vi "Vision-Target.vi"(8 "error in (no error)":errorcluster, 11 "Image Size":T5=enum."320x240") -> ()   [LabVIEW 2019]
uses:
  <vilib>/Rock Robotics/WPI/Camera/WPI_CameraImageSize.ctl
  vision/Camera Types.ctl
  <vilib>/Rock Robotics/WPI/Camera/WPI_CameraWhite Balance Values.ctl
  <vilib>/Rock Robotics/WPI/Camera/WPI_CameraExposure Values.ctl
  <vilib>/Rock Robotics/WPI/Camera/WPI_CameraFrameRate.ctl
  Robot Global Data.vi
  <vilib>/vision/NI_Vision_Development_Module.lvlib
panel:
  out "Angle":dbl
  out "Speed":dbl
  out "Possible":bool
  out "Disqualified":i32
  out "Results":T1(array[cluster]) {"Normalized Center"."x" format="%#_2g"; "Normalized Center"."y" format="%#_2g"; "Overall Score" format="%#_2g"; "Distance (ft)" format="%#_3g"; "Area Score" format="%#_2g"; "Moment Score" format="%#_2g"; "Aspect Score" format="%#_2g"}
  in  "Size Limit %":dbl=0.04 min=0.0 max=100.0 step=0.01 format="%#_13g"
  in  "Color Mode":u16(ring)=2 items=["RGB", "HSL", "HSV", "HSI"]
  in  "Particle Count":i32=5
  in  "Score Threshold %":dbl=75.0
  in  "Std Devs for Calibration":cluster{"H":dbl, "S":dbl, "V":dbl}={"H"=4.0, "S"=8.0, "V"=8.0}
  in  "Camera Type (for distance)":T2=enum."MS HD3000 square"
  in  "Annotate":bool=TRUE
  out "Qualified":i32
  in  "LED Color Range":T3={"Hue"={92.46666717529297, 124.46666717529297}, "Sat"={154.82142857142856, 255.0}, "Val"={100.17857142857144, 251.32874298095703}} {"Hue" scale=0.0..255.0 scale format="%#_3g"}
  out "Mask":T4(plugin-control)
  out "Original Image":T4(plugin-control)
  out "loop ms":u32
  out "Instructions:":string="Connect a USB or IP camera to your roboRIO. If using a ring light and retroreflective tape, use Camera Settings outside the loop create a dark image with bright and colorful stripes. If used wihtout a ring light, brighten the images so that stripes are visible.\n\nLED Color can encoded as HSL or related color modes. Calibrate to the same color as the strips being reflected to the camera. Unlike the desktop example, this LED color must be set by hand. You can also put the calibration on the dashboard and send the LED Color to the RT code using Network Tables.\n\nThe Display buttons affects whether images are displayed on the panel. It takes quite a bit of CPU  to compress and transmit the images for display.\n\nAdjust Score Cutoff to make the code more or less picky. If the color is not very unique, you may need to increase the number of particles considered. The diagram uses a Size Limit to ignore colored things that are too small. You may need to adjust it if you are targetting from far away.\n\nResults give you the distance to the target, the center and box in a normalized (-1 to 1) and pixel coordinates.\n\nBe sure to read about setting camera exposure and brightness to help simplify your image and acquire color saturated images.\n\nThere are lots of comments on the diagram to explain the code."
  # "Scores"
  # "Good target, distance ft"
  # "Bad target"
  # "Score in %"
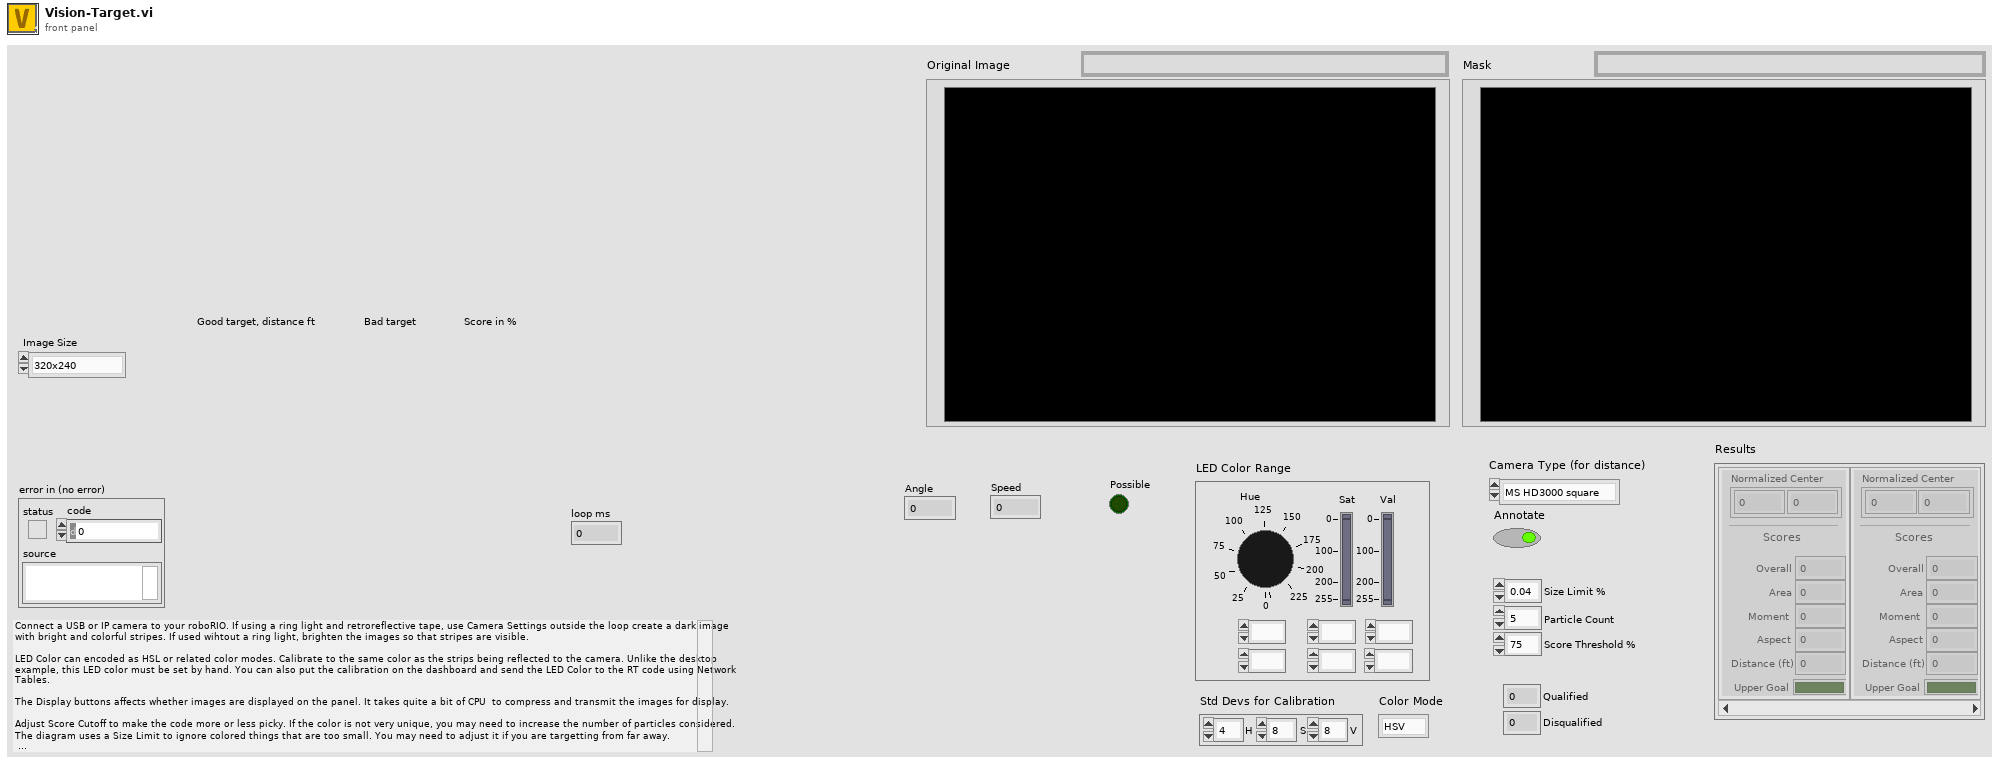
[diagram p1: front panel]
types:
  T1 = cluster{"diameter points":cluster{"first point":cluster{"x":dbl, "y":dbl}, "projected point":cluster{"x":dbl, "y":dbl}}, "Normalized Center":cluster{"x":dbl, "y":dbl}, "Overall Score":dbl, "Area Score":dbl, "Moment Score":dbl, "Aspect Score":dbl, "Distance (ft)":dbl, "Upper Goal":bool}[]
  T2 = typedef "Camera Types.ctl" = enum16{"206", "1011", "1013", "MS HD3000 square", "MS HD3000 640x480"}
  T3 = cluster{"Hue":cluster{dbl, dbl}, "Sat":cluster{dbl, dbl}, "Val":cluster{dbl, dbl}}
  T4 = typedef "IMAQ Image.ctl" = refnum<image>
  T5 = typedef "WPI_CameraImageSize.ctl" = enum16{"640x480", "320x240", "160x120", "Custom"}
  T6 = typedef "Particle Parameters" = i32
  T7 = typedef "WPI_CameraFrameRate.ctl" = u32
  T8 = typedef "WPI_CameraExposure Values.ctl" = enum16{"Auto", "Flicker-free 50 Hz", "Flicker-free 60 Hz", "Hold current", "Custom"}
  T9 = typedef "WPI_CameraWhite Balance Values.ctl" = enum16{"Auto", "Fixed indoor", "Fixed outdoor 1", "Fixed outdoor 2", "Fixed fluorescent 1", "Fixed fluorescent 2", "Hold current", "Custom"}
  T10 = typedef "Image Type" = u32
  T11 = typedef "WPI_CameraDevRef.ctl" = cluster{"Camera Address":string, "CameraStatus":errorcluster}
  T12 = enum32{"AutoM", "Close", "Dilate", "Erode", "Gradient", "Gradient out", "Gradient in", "Hit miss", "Open", "PClose", "POpen", "Thick", "Thin"}
  T13 = cluster{cluster{dbl, dbl}, cluster{dbl, dbl}, cluster{dbl, dbl}}
  T14 = cluster{"remainder":i32, "size":bool, "count":bool}
  T15 = typedef "Target Fields.ctl" = cluster{"diameter points":cluster{"first point":cluster{"x":dbl, "y":dbl}, "projected point":cluster{"x":dbl, "y":dbl}}, "normalized center":cluster{"x":dbl, "y":dbl}, "Overall Score":dbl, "Area Score":dbl, "Moment Score":dbl, "Aspect Score":dbl, "Distance (ft)":dbl, "Upper Goal":bool}
  T16 = cluster{"[0]":T15, "[1]":T15, "[2]":T15, "[3]":T15, "[4]":T15, "[5]":T15, "[6]":T15, "[7]":T15, "[8]":T15}
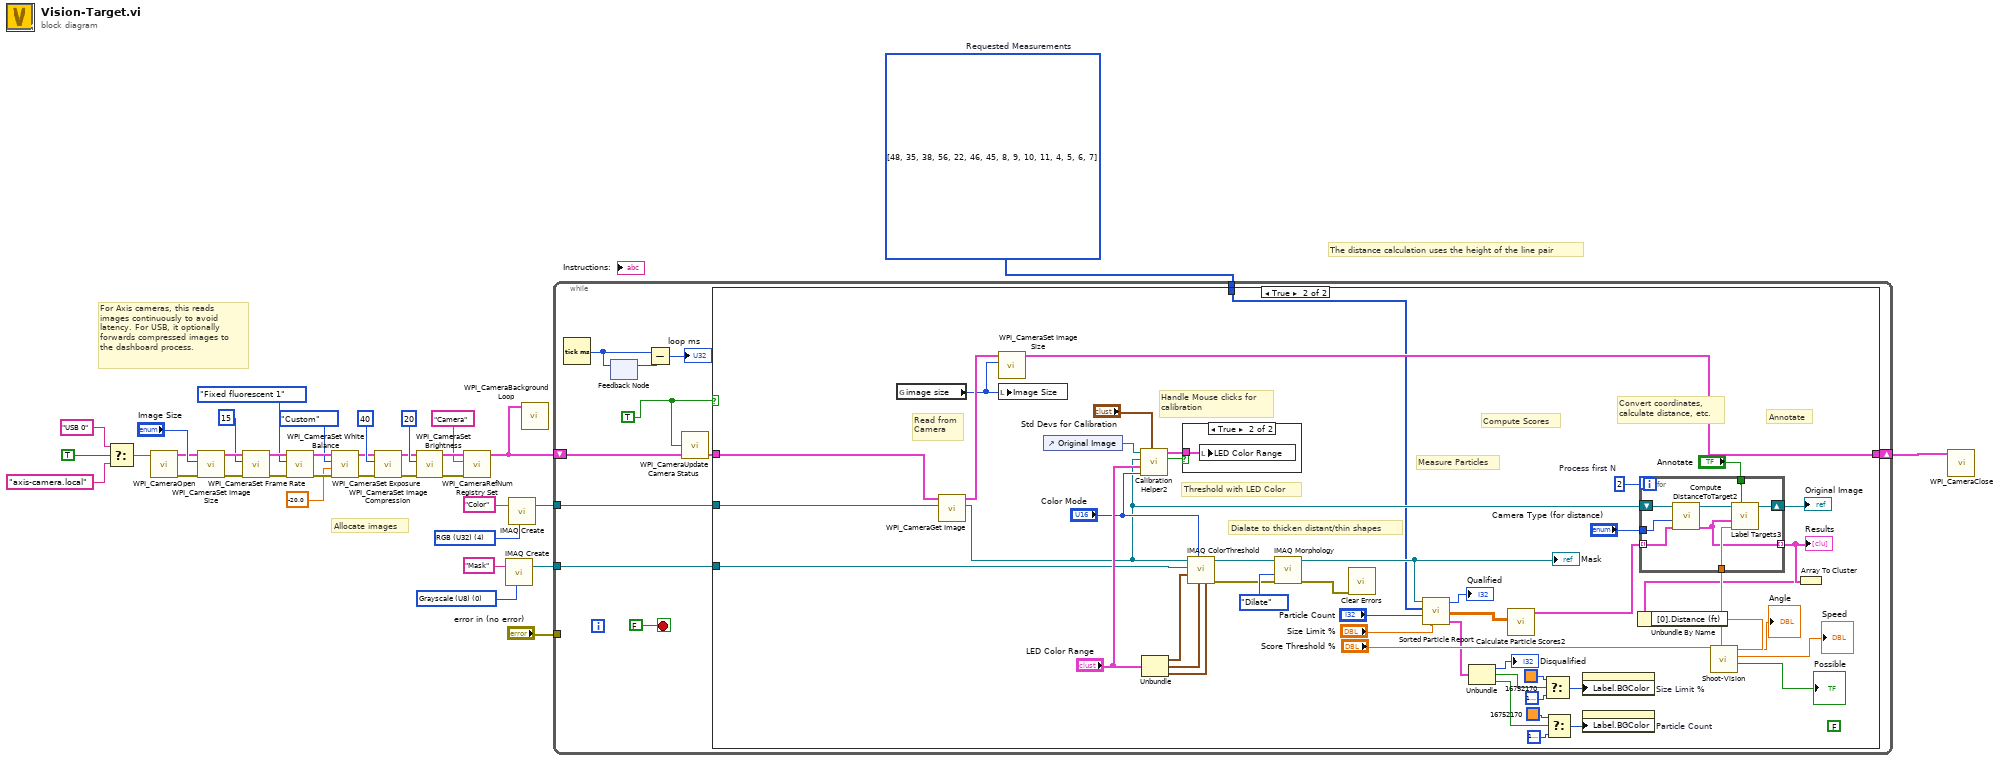
[diagram p0: block diagram]
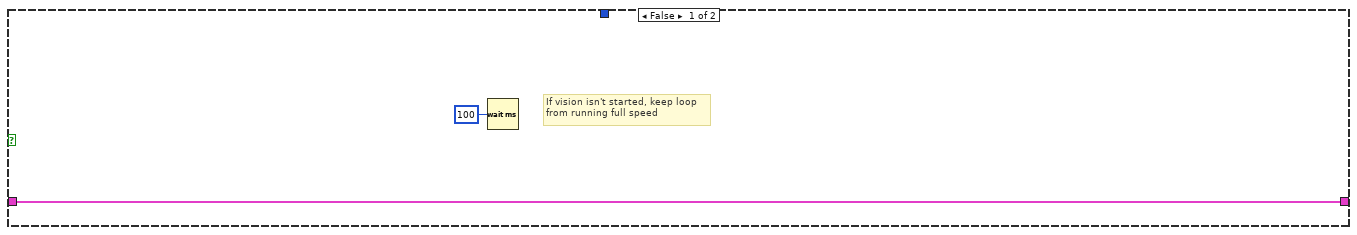
[diagram p2: hidden frame]
diagram:
  w1 = T6[] [48, 35, 38, 56, 22, 46, 45, 8, 9, 10, 11, 4, 5, 6, 7] items=["Center of Mass X", "Center of Mass Y", "First Pixel X", "First Pixel Y", "Bounding Rect Left", "Bounding Rect Top", "Bounding Rect Right", "Bounding Rect Bottom", "Max Feret Diameter Start X", "Max Feret Diameter Start Y", "Max Feret Diameter End X", "Max Feret Diameter End Y", "Max Horiz. Segment Length Left", "Max Horiz. Segment Length Right", "Max Horiz. Segment Length Row", "-", "Bounding Rect Width", "Bounding Rect Height", "Bounding Rect Diagonal", "Perimeter", "Convex Hull Perimeter", "Holes' Perimeter", "Max Feret Diameter", "Equivalent Ellipse Major Axis", "Equivalent Ellipse Minor Axis", "Equivalent Ellipse Minor Axis (Feret)", "Equivalent Rect Long Side", "Equivalent Rect Short Side", "Equivalent Rect Diagonal", "Equivalent Rect Short Side (Feret)", "Average Horiz. Segment Length", "Average Vert. Segment Length", "Hydraulic Radius", "Waddel Disk Diameter", "-", "Area", "Holes' Area", "Particle & Holes' Area", "Convex Hull Area", "Image Area", "-", "Number of Holes", "Number of Horiz. Segments", "Number of Vert. Segments", "-", "Orientation", "Max Feret Diameter Orientation", "-", "% Area/Image Area", "% Area/(Particle & Holes' Area)", "Ratio of Equivalent Ellipse Axes", "Ratio of Equivalent Rect Sides", "-", "Elongation Factor", "Compactness Factor", "Heywood Circularity Factor", "Type Factor", "-", "Sum X", "Sum Y", "Sum XX", "Sum XY", "Sum YY", "Sum XXX", "Sum XXY", "Sum XYY", "Sum YYY", "-", "Moment of Inertia XX", "Moment of Inertia XY", "Moment of Inertia YY", "Moment of Inertia XXX", "Moment of Inertia XXY", "Moment of Inertia XYY", "Moment of Inertia YYY", "Norm. Moment of Inertia XX", "Norm. Moment of Inertia XY", "Norm. Moment of Inertia YY", "Norm. Moment of Inertia XXX", "Norm. Moment of Inertia XXY", "Norm. Moment of Inertia XYY", "Norm. Moment of Inertia YYY", "Hu Moment 1", "Hu Moment 2", "Hu Moment 3", "Hu Moment 4", "Hu Moment 5", "Hu Moment 6", "Hu Moment 7"]  # Requested Measurements
  w34 = T10 0 items=["Grayscale (U8)", "Grayscale (I16)", "Grayscale (SGL)", "Complex (CSG)", "RGB (U32)", "HSL (U32)", "RGB (U64)", "Grayscale (U16)"] ("Image Type")
  w35 = T10 4 items=["Grayscale (U8)", "Grayscale (I16)", "Grayscale (SGL)", "Complex (CSG)", "RGB (U32)", "HSL (U32)", "RGB (U64)", "Grayscale (U16)"] ("Image Type")
  # "For Axis cameras, this reads\nimages continuously to avoid\nlatency. For USB, it optionally\nforwards compressed images to\nthe dashboard process."
  # "The distance calculation uses the height of the line pair"
  # "Allocate images"
  n1 = Select(t="USB 0" ("format string"), s=TRUE ("dot notation? (F)"), f="axis-camera.local" ("format string")) -> (s? t:f=w6:string)
  n2 = call <vilib>:"WPI_CameraOpen.vi"("Camera Address"=w6) -> ("error out"=w18:errorcluster, "CameraDevRef"=w19:T11)  [unwired: 1 in, 8 out]
  n3 = call <vilib>:"WPI_CameraSet Image Size.vi"("error in (no error)"=w18, "Image Size"="Image Size", "CameraDevRef"=w19) -> ("error out"=w17:errorcluster, "CameraDevRef Out"=w20:T11)  [unwired: 1 in, 6 out]
  n4 = call <vilib>:"WPI_CameraSet Frame Rate.vi"("error in (no error)"=w17, "Frame Rate (fps)"=T7 15, "CameraDevRef"=w20) -> ("error out"=w16:errorcluster, "CameraDevRef Out"=w22:T11)  [unwired: 7 out]
  n5 = call <vilib>:"WPI_CameraSet White Balance.vi"("error in (no error)"=w16, "White Balance"=WPI_CameraWhite_Balance_Values."Fixed fluorescent 1", "CameraDevRef"=w22) -> ("error out"=w15:errorcluster, "CameraDevRef Out"=w21:T11)  [unwired: 1 in, 6 out]
  n6 = call <vilib>:"WPI_CameraSet Exposure.vi"("error in (no error)"=w15, "Exposure (%)"=-20.0, "Exposure"=WPI_CameraExposure_Values."Custom", "CameraDevRef"=w21) -> ("error out"=w14:errorcluster, "CameraDevRef Out"=w24:T11)  [unwired: 6 out]
  n7 = call <vilib>:"WPI_CameraSet Image Compression.vi"("error in (no error)"=w14, "Compression"=40, "CameraDevRef"=w24) -> ("error out"=w13:errorcluster, "CameraDevRef Out"=w23:T11)  [unwired: 7 out]
  n8 = call <vilib>:"WPI_CameraSet Brightness.vi"("error in (no error)"=w13, "Brightness"=20, "CameraDevRef"=w23) -> ("error out"=w12:errorcluster, "CameraDevRef Out"=w30:T11)  [unwired: 1 in, 6 out]
  n9 = call <vilib>:"WPI_CameraRefNum Registry Set.vi"("error in (no error)"=w12, "refnum name"="Camera", "CameraDevRef"=w30) -> ("CameraDevRef"=w5:T11)  [unwired: 1 in, 7 out]
  n10 = call "IMAQ Create"("Image Name"="Mask", "Image Type"=w34) -> ("New Image"=w32:T4)  [unwired: 2 in, 2 out]
  n11 = call "IMAQ Create"("Image Name"="Color", "Image Type"=w35) -> ("New Image"=w31:T4)  [unwired: 2 in, 2 out]
  n12 = call <vilib>:"WPI_CameraBackground Loop.vi"("CameraDevRef"=w5) -> ()  [unwired: 11 in]
  n13 = while {
    tunnel: w31 -> [w44]
    tunnel: w32 -> [w46]
    tunnel: w1 -> [w45]
    shift-right: [w43] -> w4
    shift-left: w5 -> [w42]
    tunnel: "error in (no error)" -> [_]
    stop <- FALSE stop-if-true
    w37 = TRUE
    n14 = Tick Count (ms)() -> (millisecond timer value=w39:u32)
    n15 = feedback #1() -> (w40:u32)  [unwired: 1 in]
    n16 = feedback-in #1(w39) -> ()
    n17 = Subtract(x=w39, y=w40) -> (x-y=→"loop ms":u32)
    n18 = call <vilib>:"WPI_CameraUpdate Camera Status.vi"("CameraDevRef In"=w42, "Enable Vision"=w37) -> ("CameraDevRef Out"=w41:T11)  [unwired: 3 in]
    n19 = case shown="True" w37 {
      tunnel: w46 -> [_ w56]
      tunnel: w45 -> [_ w57]
      tunnel: w41 -> [w49 w97]
      tunnel: w44 -> [_ w96]
      tunnel: [w49 w93] -> w43
      frame False {
        # "If vision isn't started, keep loop\nfrom running full speed"
        n20 = Wait (ms)(milliseconds to wait=u32 100) -> ()  [unwired: 1 out]
      }
      frame True {
        w77 = 2  # Process first N
        (unwired) FALSE
        # "Dialate to thicken distant/thin shapes"
        # "Handle Mouse clicks for\ncalibration"
        # "Measure Particles"
        # "Convert coordinates,\ncalculate distance, etc."
        # "Annotate"
        # "Compute Scores"
        # "Threshold with LED Color"
        # "Read from\nCamera"
        n21 = global read "Robot Global Data.vi" "image size"() -> (w94:T5)
        n22 = call <vilib>:"WPI_CameraGet Image.vi"("Image"=w96, "CameraDevRef"=w97) -> ("Image Out"=w58:T4, "CameraDevRef Out"=w95:T11)  [unwired: 7 in, 1 out]
        n23 = call <vilib>:"WPI_CameraSet Image Size.vi"("Image Size"=w94, "CameraDevRef"=w95) -> ("CameraDevRef Out"=w93:T11)  [unwired: 2 in, 7 out]
        n24 = local write "Image Size"(w94) -> ()
        n25 = control-ref of="Original Image"() -> (w87:refnum<vi>)
        n26 = call "Calibration Helper2.vi"("Std Devs"="Std Devs for Calibration", "Color Mode"="Color Mode", "Color Components"="LED Color Range", "Image"=w58, "Image Ctl Refnum"=w87) -> ("Changed"=w86:bool, "output color"=w85:T13)  [unwired: 5 in]
        n27 = Unbundle("LED Color Range") -> ("Hue"=w92:cluster{dbl, dbl}, "Sat"=w91:cluster{dbl, dbl}, "Val"=w90:cluster{dbl, dbl})
        n28 = case shown="True" w86 {
          tunnel: w85 -> [_ w106]
          frame False {
          }
          frame True {
            n29 = local write "LED Color Range"(w106) -> ()
          }
        }
        n30 = call "IMAQ ColorThreshold"("Blue or Luma or Val or Inten Range"=w90, "Green or Sat Range"=w91, "Color Mode"="Color Mode", "Red or Hue Range"=w92, "Image Dst"=w56, "Image Src"=w58) -> ("error out"=w74:errorcluster, "Image Dst Out"=w76:T4)  [unwired: 4 in]
        n31 = call "IMAQ Morphology"("error in (no error)"=w74, "Operation"=T12."Dilate", "Image Src"=w76) -> ("error out"=w73:errorcluster, "Image Dst Out"=w70:T4)  [unwired: 7 in]
        "Mask" <- w70
        n32 = call <vilib>:"Clear Errors.vi"("error in (no error)"=w73) -> ()  [unwired: 5 in, 2 out]
        n33 = call "Sorted Particle Report.vi"("Min Area Size %"="Size Limit %", "Particle Count Limit"="Particle Count", "Pixel Measurements"=w57, "Image in"=w70) -> ("limits"=w68:T14, "Sorted Data"=w72:dbl[][], "Particles"=→"Qualified":i32)
        n34 = Unbundle(w68) -> ("remainder"=→"Disqualified":i32, "size"=w62:bool, "count"=w61:bool)
        n35 = call "Calculate Particle Scores2.vi"("Sorted Data"=w72) -> ("Scores"=w71:T15[])  [unwired: 10 in]
        n36 = Select(t=u32 16752170 ("Color"), s=w62, f=u32 16777216 ("Color")) -> (s? t:f=w60:u32)
        n37 = Select(t=u32 16752170 ("Color"), s=w61, f=u32 16777216 ("Color")) -> (s? t:f=w59:u32)
        n38 = property on="Size Limit %" class="DigNum (strict)"("Label.BGColor"=w60) -> ()  [unwired: 2 in, 2 out]
        n39 = property on="Particle Count" class="DigNum (strict)"("Label.BGColor"=w59) -> ()  [unwired: 2 in, 2 out]
        n40 = for {
          N: w77 -> [_]
          tunnel: w71 -> [w103] mode=indexing
          tunnel: "Camera Type (for distance)" -> [w105]
          tunnel: "Annotate" -> [w100]
          shift-right: [w104] -> w78
          shift-left: w58 -> [w102]
          tunnel: "Score Threshold %" -> [w99]
          tunnel: [w98] -> w54 mode=indexing
          n41 = call "Compute DistanceToTarget2.vi"("results"=w103, "Camera Type"=w105, "Image Src"=w102) -> ("results out"=w98:T15, "Image Dst Out"=w101:T4)  [unwired: 7 in]
          n42 = call "Label Targets3.vi"("Annotate"=w100, "Score Threshold"=w99, "results"=w98, "Image in"=w101) -> ("Image out"=w104:T4)  [unwired: 7 in]
        }
        "Original Image" <- w78
        "Results" <- w54
        n43 = Array To Cluster(array=w54) -> (cluster=w53:T16)
        n44 = Unbundle By Name(w53) -> ("[0].Distance (ft)"=w52:dbl)
        n45 = call "Shoot-Vision.vi"("VisionDistance"=w52) -> ("Possible"=→"Possible":bool, "Speed"=→"Speed":dbl, "Angle"=→"Angle":dbl)  [unwired: 8 in]
      }
    }
  }
  n46 = call <vilib>:"WPI_CameraClose.vi"("CameraDevRef"=w4) -> ()  [unwired: 1 in, 10 out]
